vi "FPGA Watchdog Handler.vi"   [LabVIEW 2023]
uses:
  <vilib>/rvi/Emulation/niFpgaGetClockAttributes.vi
  <vilib>/rvi/Emulation/niFpgaSctlEmulationGetInTimedLoop.vi
  <vilib>/rvi/Emulation/niFpgaEmulationReportErrorSimple.vi
  Front Panel Globals.vi
  <vilib>/rvi/eio/common/nirviEmuTemplateMethod_errors.vi
  <vilib>/rvi/Emulation/niFpgaProcessEmulError.vi
  <vilib>/rvi/Emulation/niFpgaCriticalErrorInLSC.vi
  <vilib>/eio/EIONode/EIONode.xnode
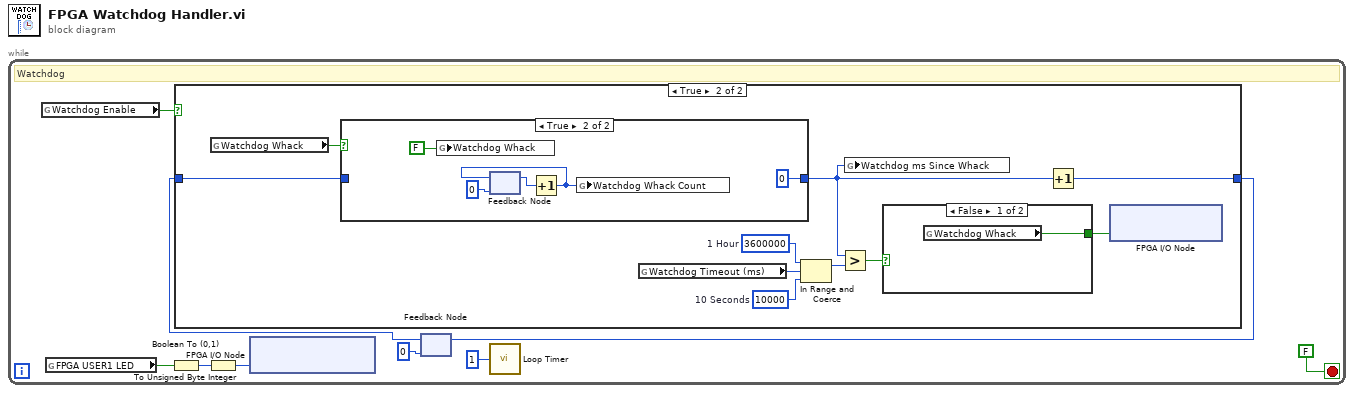
[diagram p0: block diagram]
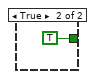
[diagram p4: hidden frame]
diagram:
  n1 = while {
    stop <- FALSE stop-if-true
    # "Watchdog"
    n2 = global read "Front Panel Globals.vi" "Watchdog Enable"() -> (w2:bool)
    n3 = global read "Front Panel Globals.vi" "FPGA USER1 LED"() -> (w1:bool)
    n4 = Boolean To (0,1)(Boolean=w1) -> (0, 1=w4:i16)
    n5 = To Unsigned Byte Integer(number=w4) -> (unsigned 8bit integer=w3:u8)
    n6 = xnode "FPGA I/O Node"("USER FPGA LED"=w3) -> ()  [unwired: 1 in, 1 out]
    n7 = feedback #1(u32 0 ("x")) -> (w8:u32)
    n8 = case shown="True" w2 {
      tunnel: [w10 w19] -> w6
      tunnel: w8 -> [w10 w18]
      frame False {
      }
      frame True {
        w15 = u32 3600000  # 1 Hour
        w16 = u32 10000  # 10 Seconds
        n9 = global read "Front Panel Globals.vi" "Watchdog Whack"() -> (w13:bool)
        n10 = case shown="True" w13 {
          tunnel: w18 -> [w21 _]
          tunnel: [w21 u32 0 ("x")] -> w12
          frame False {
          }
          frame True {
            n11 = global write "Front Panel Globals.vi" "Watchdog Whack"(FALSE ("Whack")) -> ()
            n12 = feedback #2(u32 0) -> (w24:u32)
            n13 = Increment(x=w24) -> (x+1=w23:u32)
            n14 = feedback-in #2(w23) -> ()
            n15 = global write "Front Panel Globals.vi" "Watchdog Whack Count"(w23) -> ()
          }
        }
        n16 = global read "Front Panel Globals.vi" "Watchdog Timeout (ms)"() -> (w11:u32)
        n17 = In Range and Coerce(upper limit=w15, x=w11, lower limit=w16) -> (coerced(x)=w14:u32)  [unwired: 1 out]
        n18 = Greater?(x=w12, y=w14) -> (0:w20:bool)
        n19 = global write "Front Panel Globals.vi" "Watchdog ms Since Whack"(w12) -> ()
        n20 = case shown="False" w20 {
          tunnel: [w27 TRUE ("System Reset")] -> w17
          frame False {
            n21 = global read "Front Panel Globals.vi" "Watchdog Whack"() -> (w27:bool)
          }
          frame True {
          }
        }
        n22 = Increment(x=w12) -> (x+1=w19:u32)
        n23 = xnode "FPGA I/O Node"("System Reset"=w17) -> ()  [unwired: 1 in, 1 out]
      }
    }
    n24 = feedback-in #1(w6) -> ()
    n25 = call "Loop Timer"("Count(mSec)"=u32 1) -> ()  [unwired: 1 out]
  }
